vi "setMessage.vi"(8 "error in (no error)":errorcluster, 10 "Message":string, 11 "Instance In":refnum<data-value>) -> (0 "error out":errorcluster, 3 "Instance out":refnum<data-value>)   [LabVIEW 2018, in "SingleObject.lvclass"]
uses:
  SingleObject.lvclass
  SingleObject.lvclass/SingleObject.ctl
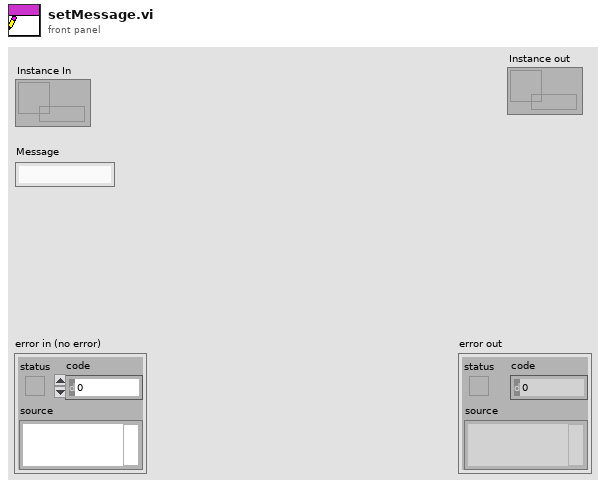
[diagram p1: front panel]
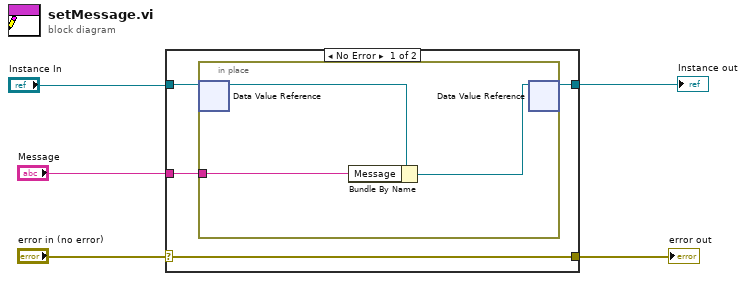
[diagram p0: block diagram]
diagram:
  n1 = case shown="No Error" "error in (no error)" {
    selector: "error in (no error)" -> [w9 w13]
    tunnel: [w9 w13] -> w4
    tunnel: [w6 w14] -> w2
    tunnel: "Instance In" -> [w7 w14]
    tunnel: "Message" -> [w8 _]
    frame No Error {
      n2 = in-place {
        in-place-border: w8 -> [w12]
        n3 = in-place-dvr #1(w7) -> (w11:refnum<class "SingleObject.lvclass">)  [unwired: 1 out]
        n4 = Bundle By Name(cluster=w11, "Message"=w12) -> (w10:refnum<class "SingleObject.lvclass">)
        n5 = in-place-dvr #1(w10) -> (w6:refnum<data-value>)  [unwired: 1 out]
      }
    }
    frame Error {
    }
  }
  "error out" <- w4
  "Instance out" <- w2
